vi "HEWH RLT Extract Channels.vi"(8 "Error In":errorcluster, 11 "Agilent Labels_Channels":T1[](array[typedef])) -> (0 "Error Out":errorcluster, 2 "Channels":string[][](array[string]), 3 "Lables":string[](array[string]))   [LabVIEW 2016]
uses:
  Type Definitions/HEWH Label Channel.ctl
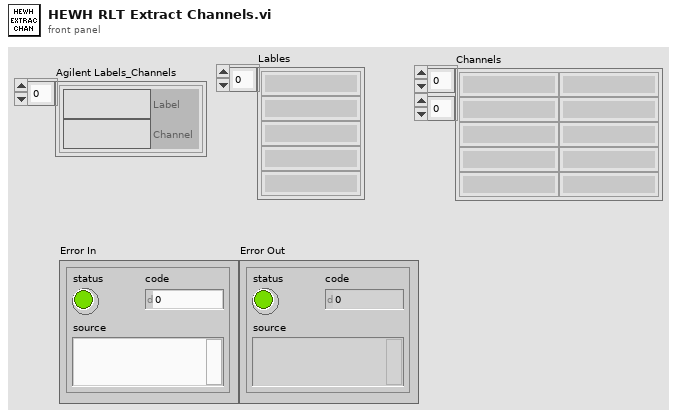
[diagram p1: front panel]
types:
  T1 = typedef "HEWH Label Channel.ctl" = cluster{"Label":string, "Channel":string}
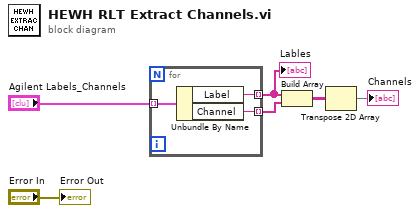
[diagram p0: block diagram]
diagram:
  n1 = for {
    tunnel: "Agilent Labels_Channels" -> [w9] mode=indexing
    tunnel: [w8] -> w3 mode=indexing
    tunnel: [w7] -> w4 mode=indexing
    n2 = Unbundle By Name(w9) -> ("Label"=w8:string, "Channel"=w7:string)
  }
  "Lables" <- w3
  n3 = Build Array(w3, w4) -> (w5:string[][])
  n4 = Transpose 2D Array(2D array=w5) -> (transposed array=→"Channels":string[][])
  "Error Out" <- "Error In"
